vi "DAQ Read.vi"(8 "error in":errorcluster, 11 "Message Data":variant) -> (0 "error out":errorcluster)   [LabVIEW 2016, in "DAQ.lvlib"]
uses:
  DAQ.lvlib
  support/Message Queue/Message Queue.lvlib
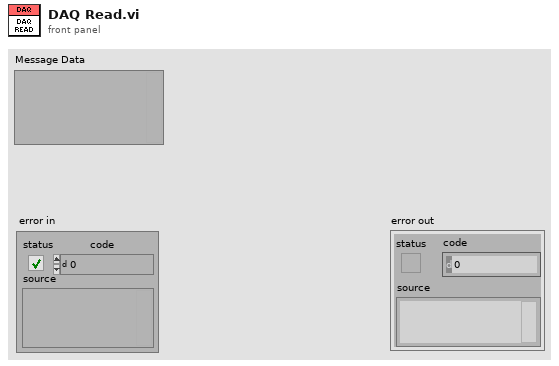
[diagram p1: front panel]
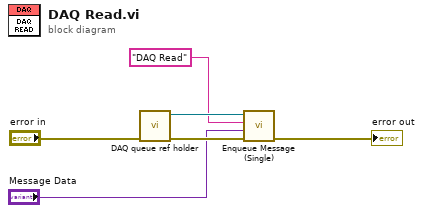
[diagram p0: block diagram]
diagram:
  n1 = call "DAQ queue ref holder.vi"("error in"="error in") -> ("error out"=w6:errorcluster, "Input Message Queue"=w3:refnum<queue>)  [unwired: 9 in]
  n2 = call "Enqueue Message (Single).vi"("error in (no error)"=w6, "Message Data"="Message Data", "Message"="DAQ Read", "Message Queue"=w3) -> ("error out"=→"error out":errorcluster)  [unwired: 6 in, 1 out]
